vi "ReceiveInferenceResults.vi"(8 "error in (no error)":errorcluster, 10 "Json Result":string, 11 "TopLevel in":refnum<class "TopLevel.lvclass">) -> (0 "error out":errorcluster, 3 "TopLevel out":refnum<class "TopLevel.lvclass">)   [LabVIEW 2019, in "TopLevel.lvlib" / "TopLevel.lvclass"]
uses:
  TopLevel.lvclass
  TopLevel.lvclass/TopLevel.ctl
  Models/InferenceResultsModel.ctl
  <vilib>/Utility/miscctls.llb/LVMapReplaceAction.ctl
  Models/ImageResultModel.ctl
  WebSocket/WebSocket Messages/UpadteImage Msg/UpdateImage Msg.lvclass/UpdateImage Msg.ctl
  <vilib>/ActorFramework/Message Enqueuer/Message Enqueuer.lvclass/Message Enqueuer.ctl
  d282e61d-8936-46a8-a2eb-d4ee9ccfbdc5.vi
  d0a66a83-b537-4283-98db-e830976e7bc0.vi
  <vilib>/ActorFramework/Message Enqueuer/Enqueue.vi
  WebSocket/WebSocket Messages/UpadteImage Msg/UpdateImage Msg.lvclass
  C:/Program Files/National Instruments/LabVIEW 2019/vi.lib/ActorFramework/Message/Message.lvclass
  <vilib>/JDP Science/JSONtext/JSON text to Variant.vi
  <vilib>/JDP Science/JSONtext/Variant to JSON Text.vi
  <vilib>/ActorFramework/Message Priority Queue/Priority Enqueue.vi
  <vilib>/JDP Science/JSONtext/LVClass Serializer/JSONtext LVClass Serializer.lvclass
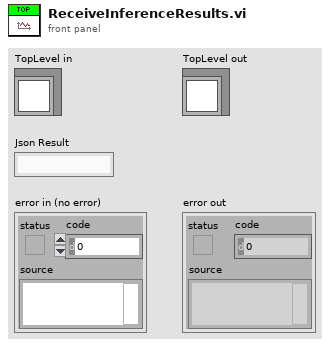
[diagram p1: front panel]
types:
  T1 = typedef "InferenceResultsModel.ctl" = cluster{"guid":string, "results":cluster{"pass":bool, "class":string}[]}
  T2 = typedef "ImageResultModel.ctl" = cluster{"image":string, "pass":bool, "class":string}
  T3 = typedef "LVMapReplaceAction.ctl" = enum32{"Modify Entry only if found", "Add or Modify Entry", "Delete Entry"}
  T4 = typedef "TopLevel.lvlib/TopLevel.lvclass/ImageResults.ctl" = cluster{"source":cluster{"image":string, "pass":bool, "class":string}, "rois":cluster{"image":string, "pass":bool, "class":string}[]}
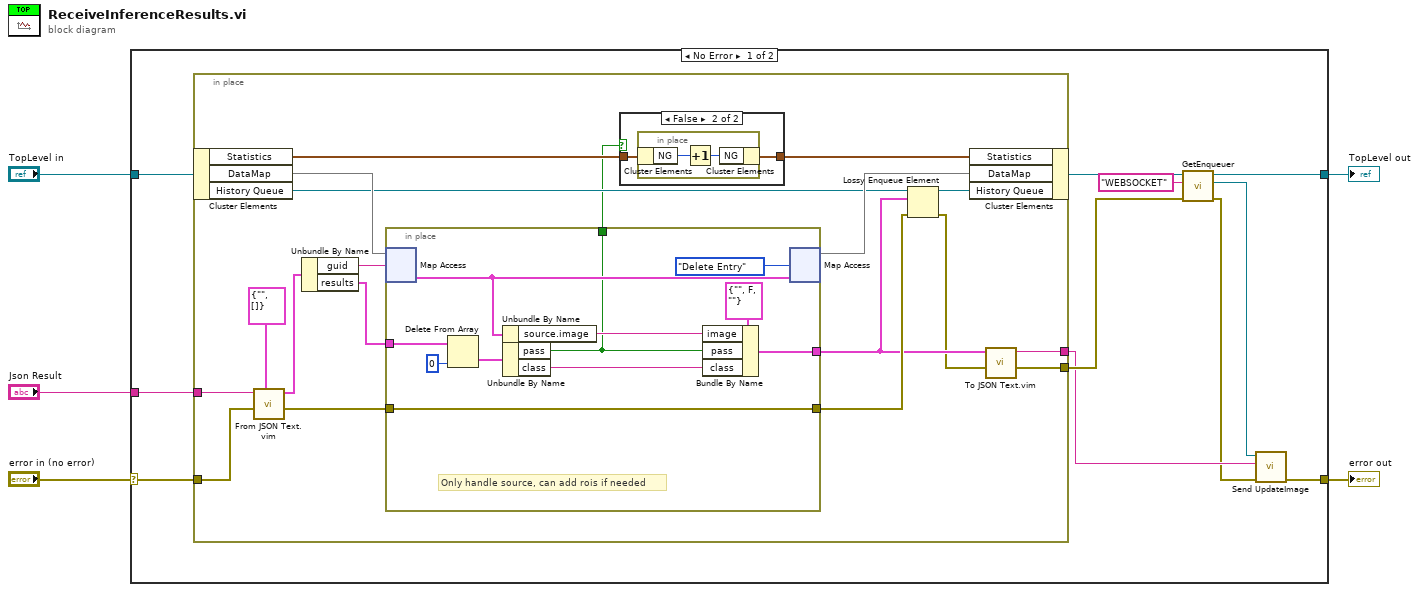
[diagram p0: block diagram]
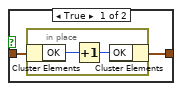
[diagram p2: hidden frame]
diagram:
  n1 = case shown="No Error" "error in (no error)" {
    selector: "error in (no error)" -> [w14 w56]
    tunnel: [w6 w56] -> w4
    tunnel: [w10 w55] -> w2
    tunnel: "TopLevel in" -> [w16 w55]
    tunnel: "Json Result" -> [w15 _]
    frame No Error {
      n2 = in-place {
        in-place-border: w15 -> [w35]
        in-place-border: w14 -> [w33]
        in-place-border: [w21] -> w12
        in-place-border: [w20] -> w8
        n3 = in-place-cluster #1(w16) -> ("Statistics"=w19:cluster{"OK":i32, "NG":i32}, "DataMap"=w27:map{string, T4}, "History Queue"=w26:refnum<queue>)
        n4 = call "From JSON Text.vim"("Data Type and Default Value"=T1 {"guid"="", "results"=[]} ("data"), "error in (no error)"=w33, "JSON"=w35) -> ("error out"=w30:errorcluster, "Data out"=w32:T1)  [unwired: 7 in]
        n5 = Unbundle By Name(w32) -> ("guid"=w31:string, "results"=w29:cluster{"pass":bool, "class":string}[])
        n6 = in-place {
          in-place-border: w30 -> [w50]
          in-place-border: w29 -> [w53]
          in-place-border: [w50] -> w24
          in-place-border: [w46] -> w23
          in-place-border: [w44] -> w17
          # "Only handle source, can add rois if needed"
          n7 = in-place-map #2(w27, w31) -> (w45:T4)  [unwired: 1 in, 1 out]
          n8 = Delete From Array(array=w53, index=0) -> (deleted portion=w51:cluster{"pass":bool, "class":string})  [unwired: 1 in, 1 out]
          n9 = Unbundle By Name(w45) -> ("source.image"=w48:string)
          n10 = Unbundle By Name(w51) -> ("pass"=w44:bool, "class"=w47:string)
          n11 = Bundle By Name(cluster=T2 {"image"="", "pass"=FALSE, "class"=""} ("element"), "image"=w48, "pass"=w44, "class"=w47) -> (w46:T2)
          n12 = in-place-map #2(w45, LVMapReplaceAction."Delete Entry" ("action")) -> (w28:map{string, T4})  [unwired: 2 out]
        }
        n13 = case shown="False" w17 {
          tunnel: w19 -> [w37 w41]
          tunnel: [w36 w40] -> w18
          frame True {
            n14 = in-place {
              n15 = in-place-cluster #3(w37) -> ("OK"=w39:i32)
              n16 = Increment(x=w39) -> (x+1=w38:i32)
              n17 = in-place-cluster #3("OK"=w38) -> (w36:cluster{"OK":i32, "NG":i32})
            }
          }
          frame False {
            n18 = in-place {
              n19 = in-place-cluster #4(w41) -> ("NG"=w43:i32)
              n20 = Increment(x=w43) -> (x+1=w42:i32)
              n21 = in-place-cluster #4("NG"=w42) -> (w40:cluster{"OK":i32, "NG":i32})
            }
          }
        }
        n22 = Lossy Enqueue Element(queue=w26, element=w23, error in (no error)=w24) -> (queue out=w25:refnum<queue>, error out=w22:errorcluster)  [unwired: 2 out]
        n23 = in-place-cluster #1("Statistics"=w18, "DataMap"=w28, "History Queue"=w25) -> (w13:refnum<class "TopLevel.lvclass">)
        n24 = call "To JSON Text.vim"("error in (no error)"=w22, "Anything"=w23) -> ("error out"=w21:errorcluster, "<JSON>"=w20:string)  [unwired: 8 in]
      }
      n25 = call "GetEnqueuer.vi"("error in (no error)"=w12, "Actor Name"="WEBSOCKET", "TopLevel in"=w13) -> ("error out"=w7:errorcluster, "Enqueuer"=w9:refnum<class "Message Enqueuer.lvclass">, "TopLevel out"=w10:refnum<class "TopLevel.lvclass">)  [unwired: 6 in]
      n26 = call "Send UpdateImage.vi"("error in (no error)"=w7, "JSON"=w8, "Message Enqueuer"=w9) -> ("error out"=w6:errorcluster)  [unwired: 7 in, 1 out]
    }
    frame Error {
    }
  }
  "error out" <- w4
  "TopLevel out" <- w2
